vi "Fibonacci.vi"(1 "Index":u32) -> (0 "Result":u32)   [LabVIEW 2019]
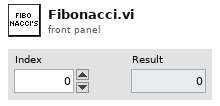
[diagram p1: front panel]
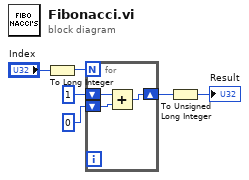
[diagram p0: block diagram]
diagram:
  n1 = To Long Integer(number="Index") -> (32bit integer=w3:i32)
  n2 = for {
    N: w3 -> [_]
    shift-right: [w7] -> w2
    shift-left: 1 -> [w9]
    shift-left: 0 -> [w8]
    n3 = Add(x=w9, y=w8) -> (x+y=w7:i32)
  }
  n4 = To Unsigned Long Integer(number=w2) -> (unsigned 32bit integer=→"Result":u32)
